vi "POLARIS Fluence Camera.vi"() -> ()   [LabVIEW 2014]
uses:
  XDisplay/POLARIS IMAQ Display.xctl
  IMAQdx Cam/IMAQdx Cam.lvclass
  XDisplay/Properties/ImageSource.ctl
  Analyze Classes/Analyze Fluence/Analyze Fluence.lvclass
  Analyze Classes/Analyze Timer/Analyze Timer.lvclass
  Utility/POLARIS Vision utility.lvlib
panel:
  in  "Camera Name":string
  in  "Config Dir":path
  in  "WorkDir":path
  in  "Prefix":string
  in  "Show settings":bool
  out "XDisplay":cluster{"Image":T1}(xcontrol)
  in  "Shot Rate (sec)":u16=50
  out "error load settings":errorcluster
  in  "stop2":bool
  out "Max Fluence J/cm2":dbl format="%#_3g"
  in  "Size of hot Region":i32=10
  in  "Energy [J]":dbl=10.0
  in  "stop":bool
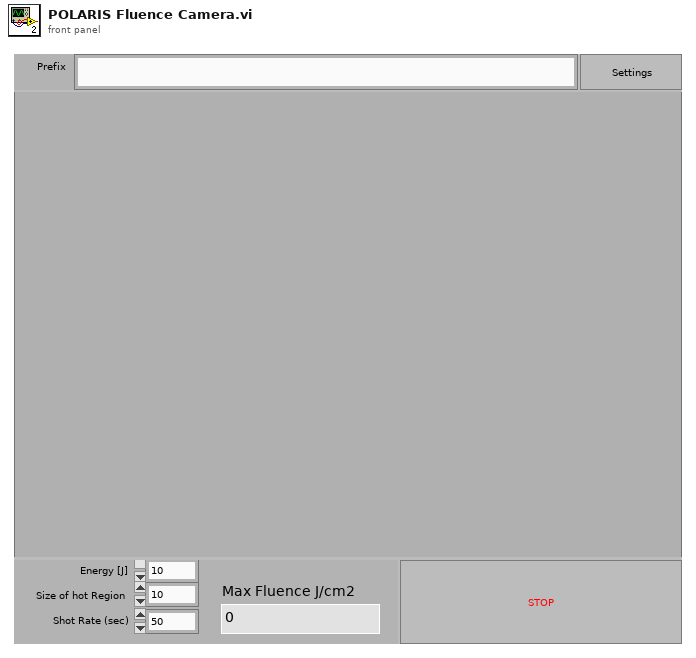
[diagram p1: front panel]
types:
  T1 = typedef "IMAQ Image.ctl" = refnum<image>
  T2 = typedef "POLARIS IMAQ Display.xctl/ImageSource.ctl" = enum16{"Camera", "File"}
  T3 = typedef "Image Type" = u32
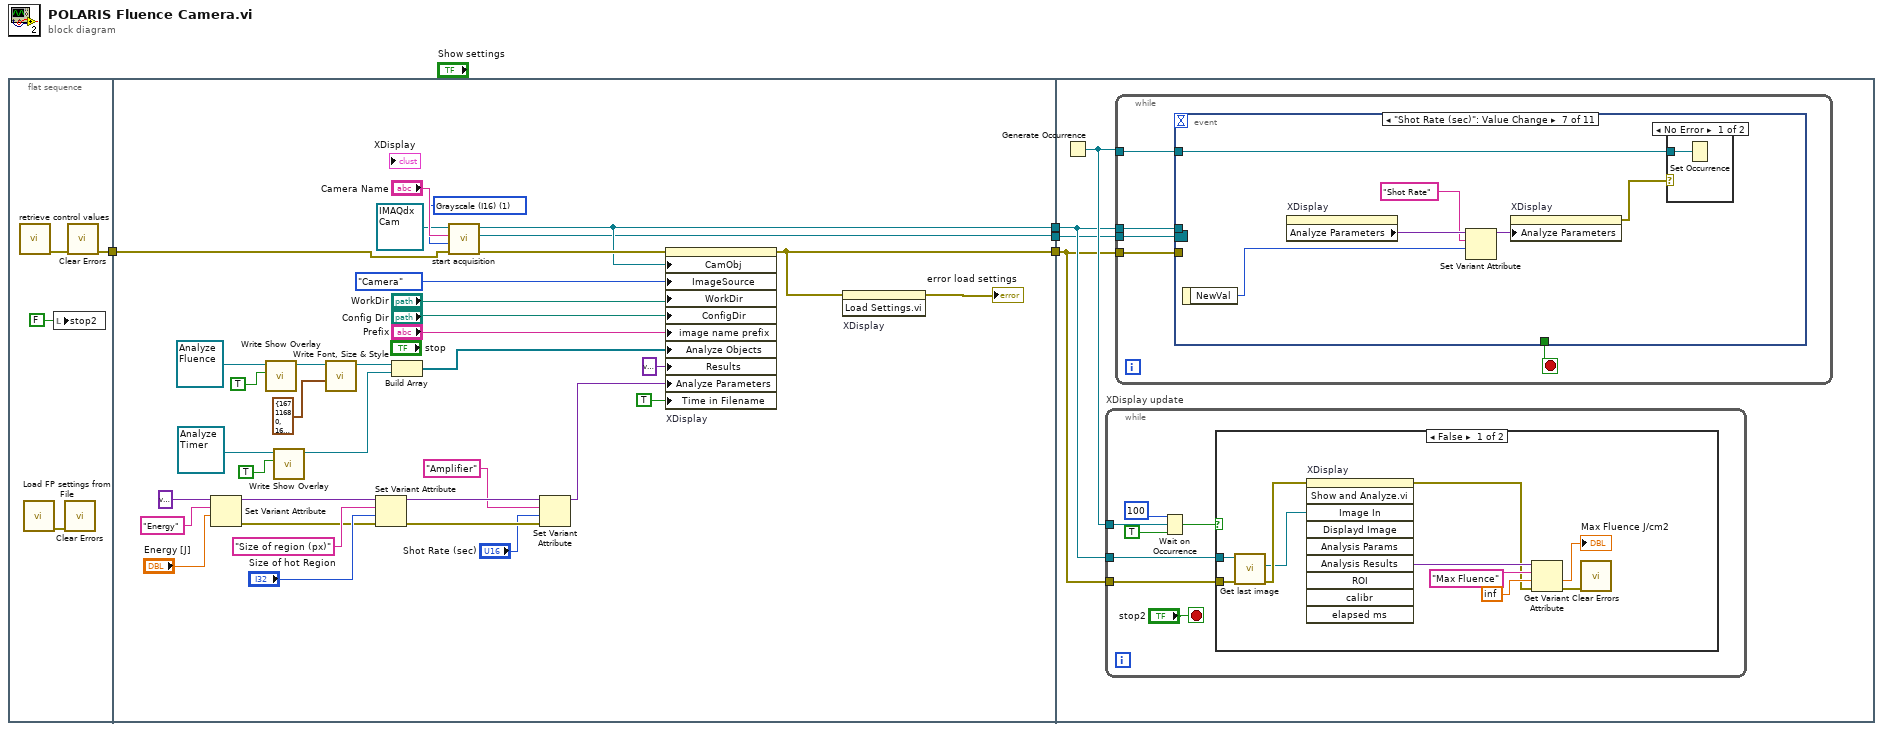
[diagram p0: block diagram]
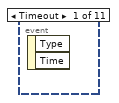
[diagram p3: hidden frame]
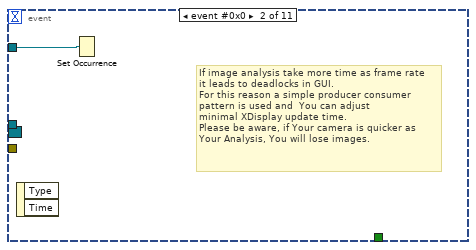
[diagram p4: hidden frame]
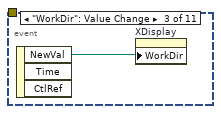
[diagram p5: hidden frame]
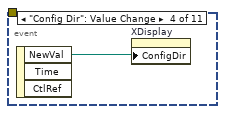
[diagram p6: hidden frame]
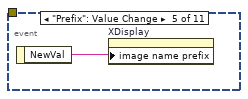
[diagram p7: hidden frame]
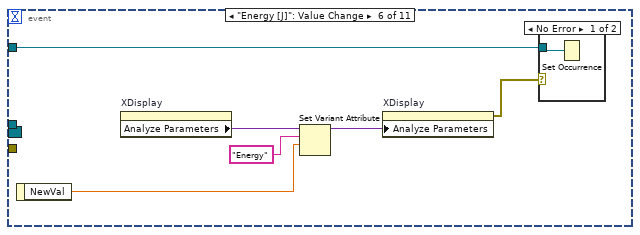
[diagram p8: hidden frame]
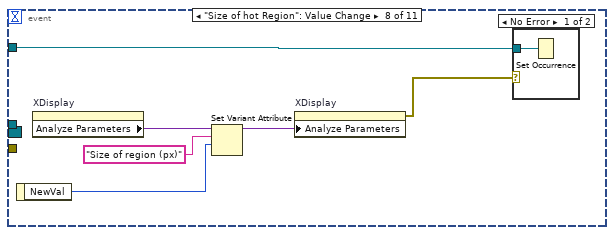
[diagram p11: hidden frame]
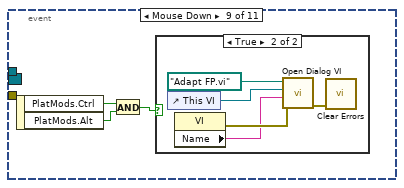
[diagram p13: hidden frame]
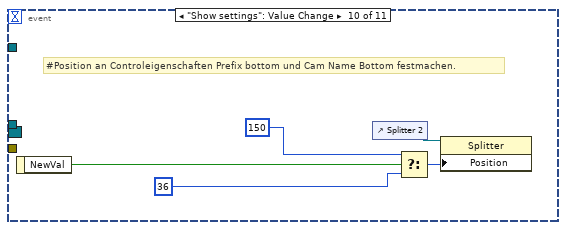
[diagram p15: hidden frame]
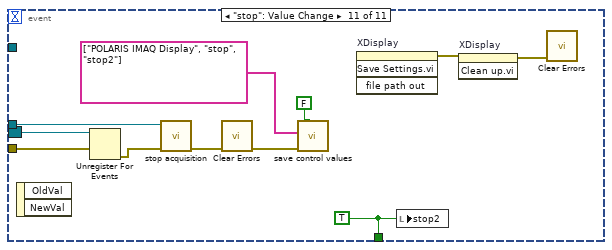
[diagram p16: hidden frame]
diagram:
  n1 = flat-sequence {
    tunnel: [w6] -> w4
    tunnel: w4 -> [w34]
    tunnel: [w19] -> w3
    tunnel: [w18] -> w2
    tunnel: [w17] -> w1
    tunnel: w3 -> [w47]
    tunnel: w2 -> [w46]
    tunnel: w1 -> [w45]
    frame #0 {
      n2 = call "retrieve control values.vi"() -> ("error out"=w7:errorcluster)  [unwired: 10 in, 1 out]
      n3 = call "Load FP settings from File.vi"() -> ("error out"=w5:errorcluster)  [unwired: 11 in]
      n4 = local write "stop2"(FALSE ("stop2")) -> ()
      n5 = call <vilib>:"Clear Errors.vi"("error in (no error)"=w5) -> ()  [unwired: 5 in, 2 out]
      n6 = call <vilib>:"Clear Errors.vi"("error in (no error)"=w7) -> ("error out"=w6:errorcluster)  [unwired: 5 in, 1 out]
    }
    frame #1 {
      w39 = T3 1 items=["Grayscale (U8)", "Grayscale (I16)", "Grayscale (SGL)", "Complex (CSG)", "RGB (U32)", "HSL (U32)", "RGB (U64)", "Grayscale (U16)"] ("Image Type")
      n7 = Set Variant Attribute(Variant=variant ("variant"), name="Energy", value="Energy [J]") -> (Variant out=w33:variant, error out=w22:errorcluster)  [unwired: 1 in, 1 out]
      n8 = call-dynamic "Write Show Overlay.vi"("Overlay?"=TRUE, "Analyze BaseClass in"=refnum<class "Analyze Fluence.lvclass"> refnum ("Analyze Fluence.lvclass")) -> ("Analyze BaseClass out"=w24:refnum<class "Analyze Fluence.lvclass">)  [unwired: 8 in, 1 out]
      n9 = call-dynamic "Write Show Overlay.vi"("Overlay?"=TRUE, "Analyze BaseClass in"=refnum<class "Analyze Timer.lvclass"> refnum ("Analyze Timer.lvclass")) -> ("Analyze BaseClass out"=w14:refnum<class "Analyze Timer.lvclass">)  [unwired: 8 in, 1 out]
      n10 = call-dynamic "Write Font, Size & Style.vi"("Overlay colors"=cluster{"Border":u32, "Text":u32} {"Border"=16711680, "Text"=16448250}, "Analyze BaseClass in"=w24) -> ("Analyze BaseClass out"=w23:refnum<class "Analyze Fluence.lvclass">)  [unwired: 8 in, 1 out]
      n11 = Set Variant Attribute(Variant=w33, name="Size of region (px)", value="Size of hot Region", error in=w22) -> (Variant out=w13:variant, error out=w11:errorcluster)  [unwired: 1 out]
      n12 = Build Array(w23, w14) -> (w35:refnum<class "Analyze BaseClass.lvclass">[])
      n13 = call-dynamic "start acquisition.vi"("error in (no error)"=w34, "Image Type"=w39, "Camera Name"="Camera Name", "IMAQdx Cam in"=refnum<class "IMAQdx Cam.lvclass"> refnum ("IMAQdx Cam.lvclass")) -> ("error out"=w40:errorcluster, "Event Registration Refnum"=w18:refnum<event-registration>, "IMAQdx Cam out"=w19:refnum<class "IMAQdx Cam.lvclass">)  [unwired: 5 in]
      n14 = Set Variant Attribute(Variant=w13, name="Amplifier", value="Shot Rate (sec)", error in=w11) -> (Variant out=w12:variant)  [unwired: 2 out]
      n15 = property on="XDisplay" class="POLARIS IMAQ Display (strict)"(error in=w40, "CamObj"=w19, "ImageSource"=ImageSource."Camera", "WorkDir"="WorkDir", "ConfigDir"="Config Dir", "image name prefix"="Prefix", "Analyze Objects"=w35, "Results"=variant, "Analyze Parameters"=w12, "Time in Filename"=TRUE) -> (error out=w17:errorcluster)  [unwired: 1 in, 1 out]
      n16 = invoke on="XDisplay" class="POLARIS IMAQ Display (strict)" method="Load Settings.vi"(error in=w17) -> (error out=→"error load settings":errorcluster)  [unwired: 2 in, 2 out]
    }
    frame #2 {
      n17 = Generate Occurrence() -> (w48:refnum<k4>)
      n18 = while "XDisplay update" {
        tunnel: w48 -> [w55]
        tunnel: w47 -> [w52]
        tunnel: w45 -> [w51]
        stop <- "stop2" stop-if-true
        n19 = Wait on Occurrence(1:TRUE ("ignore previous (T)"), 2:w55, 3:100 ("ms timeout (-1)")) -> (0:w53:bool)
        n20 = case shown="False" w53 {
          tunnel: w52 -> [w64 _]
          tunnel: w51 -> [w65 _]
          frame False {
            n21 = call-dynamic "Get last image.vi"("error in (no error)"=w65, "IMAQdx Cam in"=w64) -> ("error out"=w63:errorcluster, "Image Out"=w62:T1)  [unwired: 6 in, 2 out]
            n22 = invoke on="XDisplay" class="POLARIS IMAQ Display (strict)" method="Show and Analyze.vi"(error in=w63, "Image In"=w62) -> (error out=w57:errorcluster, "Analysis Results"=w58:variant)  [unwired: 8 in, 8 out]
            n23 = Get Variant Attribute(Variant=w58, name="Max Fluence", default value (empty Variant)=inf, error in=w57) -> (value=→"Max Fluence J/cm2":dbl, error out=w56:errorcluster)  [unwired: 2 out]
            n24 = call <vilib>:"Clear Errors.vi"("error in (no error)"=w56) -> ()  [unwired: 5 in, 2 out]
          }
          frame True {
          }
        }
      }
      n25 = while {
        tunnel: w47 -> [w69]
        tunnel: w46 -> [w68]
        tunnel: w45 -> [w67]
        tunnel: w48 -> [w66]
        stop <- w70 stop-if-true
        n26 = event shown="[6] \"Shot Rate (sec)\": Value Change" {
          selector: w68 -> [_ _ _ _ _ _ _ _ _ _ w117]
          dyn-events: _ -> [_ _ _ _ _ _ _ _ _ _ _]
          timeout: _ -> [_ _ _ _ _ _ _ _ _ _ _]
          tunnel: [_ _ _ _ _ _ _ _ _ _ w112] -> w70
          tunnel: w69 -> [_ _ _ _ _ _ _ _ _ _ w118]
          tunnel: w67 -> [_ _ _ _ _ _ _ _ _ _ w116]
          tunnel: w66 -> [_ w71 _ _ _ w75 w83 w90 _ _ _]
          event Timeout {
            n27 = event-data() -> ()  [unwired: 1 in, 2 out]
          }
          event event #0x0 {
            # "If image analysis take more time as frame rate\nit leads to deadlocks in GUI.\nFor this reason a simple producer consumer \npattern is used and  You can adjust \nminimal XDisplay update time.\nPlease be aware, if Your camera is quicker as\nYour Analysis, You will lose images."
            n28 = event-data() -> ()  [unwired: 1 in, 2 out]
            n29 = Set Occurrence(w71) -> ()
          }
          event "WorkDir": Value Change {
            n30 = event-data() -> ("NewVal"=w72:path)  [unwired: 1 in, 2 out]
            n31 = property on="XDisplay" class="POLARIS IMAQ Display (strict)"("WorkDir"=w72) -> ()  [unwired: 2 in, 2 out]
          }
          event "Config Dir": Value Change {
            n32 = event-data() -> ("NewVal"=w73:path)  [unwired: 1 in, 2 out]
            n33 = property on="XDisplay" class="POLARIS IMAQ Display (strict)"("ConfigDir"=w73) -> ()  [unwired: 2 in, 2 out]
          }
          event "Prefix": Value Change {
            n34 = event-data() -> ("NewVal"=w74:string)  [unwired: 1 in]
            n35 = property on="XDisplay" class="POLARIS IMAQ Display (strict)"("image name prefix"=w74) -> ()  [unwired: 2 in, 2 out]
          }
          event "Energy [J]": Value Change {
            n36 = event-data() -> ("NewVal"=w77:dbl)  [unwired: 1 in]
            n37 = property on="XDisplay" class="POLARIS IMAQ Display (strict)"() -> ("Analyze Parameters"=w80:variant)  [unwired: 2 in, 2 out]
            n38 = Set Variant Attribute(Variant=w80, name="Energy", value=w77) -> (Variant out=w78:variant)  [unwired: 1 in, 2 out]
            n39 = property on="XDisplay" class="POLARIS IMAQ Display (strict)"("Analyze Parameters"=w78) -> (error out=w76:errorcluster)  [unwired: 2 in, 1 out]
            n40 = case shown="No Error" w76 {
              tunnel: w75 -> [w81 _]
              frame No Error {
                n41 = Set Occurrence(w81) -> ()
              }
              frame Error {
              }
            }
          }
          event "Shot Rate (sec)": Value Change {
            n42 = event-data() -> ("NewVal"=w84:u16)  [unwired: 1 in]
            n43 = property on="XDisplay" class="POLARIS IMAQ Display (strict)"() -> ("Analyze Parameters"=w87:variant)  [unwired: 2 in, 2 out]
            n44 = Set Variant Attribute(Variant=w87, name="Shot Rate", value=w84) -> (Variant out=w86:variant)  [unwired: 1 in, 2 out]
            n45 = property on="XDisplay" class="POLARIS IMAQ Display (strict)"("Analyze Parameters"=w86) -> (error out=w82:errorcluster)  [unwired: 2 in, 1 out]
            n46 = case shown="No Error" w82 {
              tunnel: w83 -> [w88 _]
              frame No Error {
                n47 = Set Occurrence(w88) -> ()
              }
              frame Error {
              }
            }
          }
          event "Size of hot Region": Value Change {
            n48 = event-data() -> ("NewVal"=w91:i32)  [unwired: 1 in]
            n49 = property on="XDisplay" class="POLARIS IMAQ Display (strict)"() -> ("Analyze Parameters"=w94:variant)  [unwired: 2 in, 2 out]
            n50 = Set Variant Attribute(Variant=w94, name="Size of region (px)", value=w91) -> (Variant out=w92:variant)  [unwired: 1 in, 2 out]
            n51 = property on="XDisplay" class="POLARIS IMAQ Display (strict)"("Analyze Parameters"=w92) -> (error out=w89:errorcluster)  [unwired: 2 in, 1 out]
            n52 = case shown="No Error" w89 {
              tunnel: w90 -> [w95 _]
              frame No Error {
                n53 = Set Occurrence(w95) -> ()
              }
              frame Error {
              }
            }
          }
          event Mouse Down {
            n54 = event-data() -> ("PlatMods.Ctrl"=w98:bool, "PlatMods.Alt"=w96:bool)  [unwired: 1 in]
            n55 = And(x=w98, y=w96) -> (x .and. y?=w97:bool)
            n56 = case shown="True" w97 {
              frame False {
              }
              frame True {
                n57 = control-ref of="This VI"() -> (w102:refnum<vi>)
                n58 = property class="VI"() -> (error out=w101:errorcluster, "Name"=w100:string)  [unwired: 2 in, 1 out]
                n59 = call "Open Dialog VI.vi"("error in"=w101, "Windows title"=w100, "ref for signalling"=w102, "vi path"=path "Adapt FP.vi") -> ("error out"=w99:errorcluster)  [unwired: 7 in]
                n60 = call <vilib>:"Clear Errors.vi"("error in (no error)"=w99) -> ()  [unwired: 5 in, 2 out]
              }
            }
          }
          event "Show settings": Value Change {
            # "#Position an Controleigenschaften Prefix bottom und Cam Name Bottom festmachen."
            n61 = event-data() -> ("NewVal"=w107:bool)  [unwired: 1 in]
            n62 = control-ref of="Splitter 2"() -> (w108:refnum<vi>)
            n63 = Select(t=150, s=w107, f=36 ("t")) -> (s? t:f=w106:i32)
            n64 = property class="Splitter"(reference=w108, "Position"=w106) -> ()  [unwired: 1 in, 2 out]
          }
          event "stop": Value Change {
            w112 = TRUE
            n65 = event-data() -> ()  [unwired: 1 in, 2 out]
            n66 = Unregister For Events(event registration refnum=w117, error in=w116) -> (error out=w119:errorcluster)
            n67 = call-dynamic "stop acquisition.vi"("error in (no error)"=w119, "IMAQdx Cam in"=w118) -> ("error out"=w115:errorcluster)  [unwired: 8 in, 1 out]
            n68 = call <vilib>:"Clear Errors.vi"("error in (no error)"=w115) -> ("error out"=w114:errorcluster)  [unwired: 5 in, 1 out]
            n69 = call "save control values.vi"("Append timestamp (true)"=FALSE, "error in"=w114, "Dont save"=string[] ["POLARIS IMAQ Display", "stop", "stop2"]) -> ()  [unwired: 5 in, 2 out]
            n70 = invoke on="XDisplay" class="POLARIS IMAQ Display (strict)" method="Save Settings.vi"() -> (error out=w110:errorcluster)  [unwired: 4 in, 3 out]
            n71 = local write "stop2"(w112) -> ()
            n72 = invoke on="XDisplay" class="POLARIS IMAQ Display (strict)" method="Clean up.vi"(error in=w110) -> (error out=w109:errorcluster)  [unwired: 2 in, 2 out]
            n73 = call <vilib>:"Clear Errors.vi"("error in (no error)"=w109) -> ()  [unwired: 5 in, 2 out]
          }
        }
      }
    }
  }
